vi "niDTS BT BDR Rx Test Example.vi"() -> ()   [LabVIEW 2014]
uses:
  Rx Test/Includes/niDTS BT Rx Test INC Results.ctl
  BDR Rx Test/Includes/niDTS BT BDR Rx Test INC Parameters.ctl
  BDR Tx Test/Includes/niDTS BT INC BDR Packet Type.ctl
  Tx Test/Includes/niDTS BT Tx Test INC BD Payload Data.ctl
  Rx Test/Includes/niDTS BT Rx Test INC Carrier Mode.ctl
  Rx Test/Includes/niDTS BT Rx Test INC Packet Header.ctl
  Rx Test/Includes/niDTS BT Rx Test INC Payload Header.ctl
  Includes/niDTS BT DUT INC SG Trigger.ctl
  CommLib/Includes/niDTS Comm INC CLI Login.ctl
  EDR Rx Test/Includes/niDTS BT EDR Rx Test INC Parameters.ctl
  LE Rx Test/Includes/niDTS BT LE Rx Test INC Parameters.ctl
  Rx Test/Includes/niDTS BT Rx Test INC LE Payload Length.ctl
  Framework/Logger/Includes/niDTS Logger INC File Parameters.ctl
  TestStand/Station/Objects/SystemDutHandle/niDTS SystemDutHandle.lvclass
  Framework/niDTS Framework.lvlib
  TestStand/niDTS TestStand.lvlib
  Plugins/niBCM4350 BT/niBCM4350 BT.lvlib
  niDTS BT.lvlib
  Tx Test/Objects/BASE_class/niDTS BT Tx Test.lvclass
  Rx Test/Objects/BASE_class/niDTS BT Rx Test.lvclass
  Plugins/niLEDTM BT/niLEDTM BT.lvlib
  CommLib/niDTS CommLib.lvlib
panel:
  in  "Result Index":i32=1
  in  "Tab Control":enum32{"BDR", "EDR", "LE TP"}(tab)
  in  "BDR Rx Input Parameters":T1={"Channel"=0, "Tx Power (dBm) "=-70.0, "External Attenuation (dB)"=0.0, "BDR Packet type"=enum."DH1", "Payload Data"=enum."PN9", "Carrier Mode"=enum."Burst", "Number of Packets"=-1, "Report Period (ms)"=1000.0, "BD ADDRESS"="\u0000\u0000\u0000\u0000\u0000\u0000", "Packet Header"={"LT Address"=0, "Flow"=0, "ARQN"=enum."NAK", "Sequence Bit"=0}, "Dirty Packets"=FALSE, "Corrupt Alternate CRC"=FALSE, "Payload Header"={"LCh"=0, "HeaderFlowControlBit"=FALSE, "Length (-1 AutoSet Max)"=-1}, "Trigger"={"TriggerEdge"=enum."RISing", "TriggerSource"=enum."IMMediate", "TriggerDelay (sec)"=0.0, "TriggerTimeout (sec)"=0.0}}
  out "Results":T8
  out "BDR USL":T8={"Total Packets Received (LE)"=2147483647, "Packets Sent (LE)"=inf, "Good Packets"=inf, "Packet Error Rate (%)"=1.0, "Error Bits"=4294967295, "Good Bits"=4294967295, "Total Received Bits"=4294967295, "Bit Error Rate (%)"=1.0}
  out "BDR LSL":T8
  out "EDR USL":T8={"Total Packets Received (LE)"=2147483647, "Packets Sent (LE)"=inf, "Good Packets"=inf, "Packet Error Rate (%)"=1.0, "Error Bits"=4294967295, "Good Bits"=4294967295, "Total Received Bits"=4294967295, "Bit Error Rate (%)"=1.0}
  out "EDR LSL":T8
  out "EDR RX Results":T8
  in  "EDR Rx Input Parameters":T9={"Channel"=0, "Tx Power (dBm)"=-70.0, "External Attenuation (dB)"=0.0, "EDR Packet type"=enum."DH1", "Data Rate (bits/symbol)"=2, "Payload Data"=enum."PN9", "Carrier Mode"=enum."Burst", "Number of Packets"=-1, "Report Period (ms)"=1000.0, "BD ADDRESS"="\u0000\u0000\u0000\u0000\u0000\u0000", "Dirty Packets"=FALSE, "Corrupt Alternate CRC"=FALSE, "Packet Header"={"LT Address"=0, "Flow"=0, "ARQN"=enum."NAK", "Sequence Bit"=0}, "Payload Header"={"LCh"=0, "HeaderFlowControlBit"=FALSE, "Length (-1 AutoSet Max)"=-1}, "Trigger"={"TriggerEdge"=enum."RISing", "TriggerSource"=enum."IMMediate", "TriggerDelay (sec)"=0.0, "TriggerTimeout (sec)"=0.0}}
  out "LE USL":T8={"Total Packets Received (LE)"=2147483647, "Packets Sent (LE)"=inf, "Good Packets"=inf, "Packet Error Rate (%)"=1.0, "Error Bits"=4294967295, "Good Bits"=4294967295, "Total Received Bits"=4294967295, "Bit Error Rate (%)"=1.0}
  out "LE LSL":T8
  out "LE Resutls":T8={"Total Packets Received (LE)"=1500, "Packets Sent (LE)"=1500.0, "Good Packets"=0.0, "Packet Error Rate (%)"=0.0, "Error Bits"=0, "Good Bits"=0, "Total Received Bits"=0, "Bit Error Rate (%)"=0.0}
  in  "BT LE Parameters":T10={"Channel"=0, "Tx Power (dBm)"=-70.0, "External Attenuation (dB)"=0.0, "Payload Data"=enum."PN9", "Carrier Mode"=enum."Burst", "Number of Packets"=1500, "Corrupt Alternate CRC"=FALSE, "Dirty Tx"=FALSE, "Payload Header"={"Length (-1 AutoSet Max)"=-1}, "Trigger"={"TriggerEdge"=enum."RISing", "TriggerSource"=enum."IMMediate", "TriggerDelay (sec)"=0.0, "TriggerTimeout (sec)"=0.0}}
  in  "General Parameters":T13={"Port Parameters Serial"={"baud rate "=115200, "data bits"=8, "Enable Termination Char"=TRUE, "flow control"=0, "parity"=enum."None", "timeout (ms) "=5000, "stop bits"=10, "termination char"=10}, "CLI Login"={"Do Login"=FALSE, "Login Prompt"="", "Password"="", "User Name"=""}}
  in  "Socket Index":i32
  in  "System Configuration Path":path=path "C:/Users/Public/Documents/National Instruments/WTM 1.0/System Configurations/BTDev4_28_2015.xml"
  in  "DUT Plugin":enum32{"LE DTM", "BCM4350"}(tab)=enum."BCM4350"
  in  "Interfaces LE DTM":enum32{"Serial", "Other"}(tab)
  in  "Port Parameters":T14(array[cluster])=[{"BT"={"Serial Resource"="COM5"}}, {"BT"={"Serial Resource"="COM5"}}]
  in  "Interfaces BCM4350":enum32{"Serial", "Other"}(tab)
  in  "Port Parameters":T14(array[cluster])=[{"BT"={"Serial Resource"="COM5"}}, {"BT"={"Serial Resource"="COM5"}}]
  out "error out":errorcluster
  # "BD Address Order"
  # "LAP(24)UAP(8)NAP(16)"
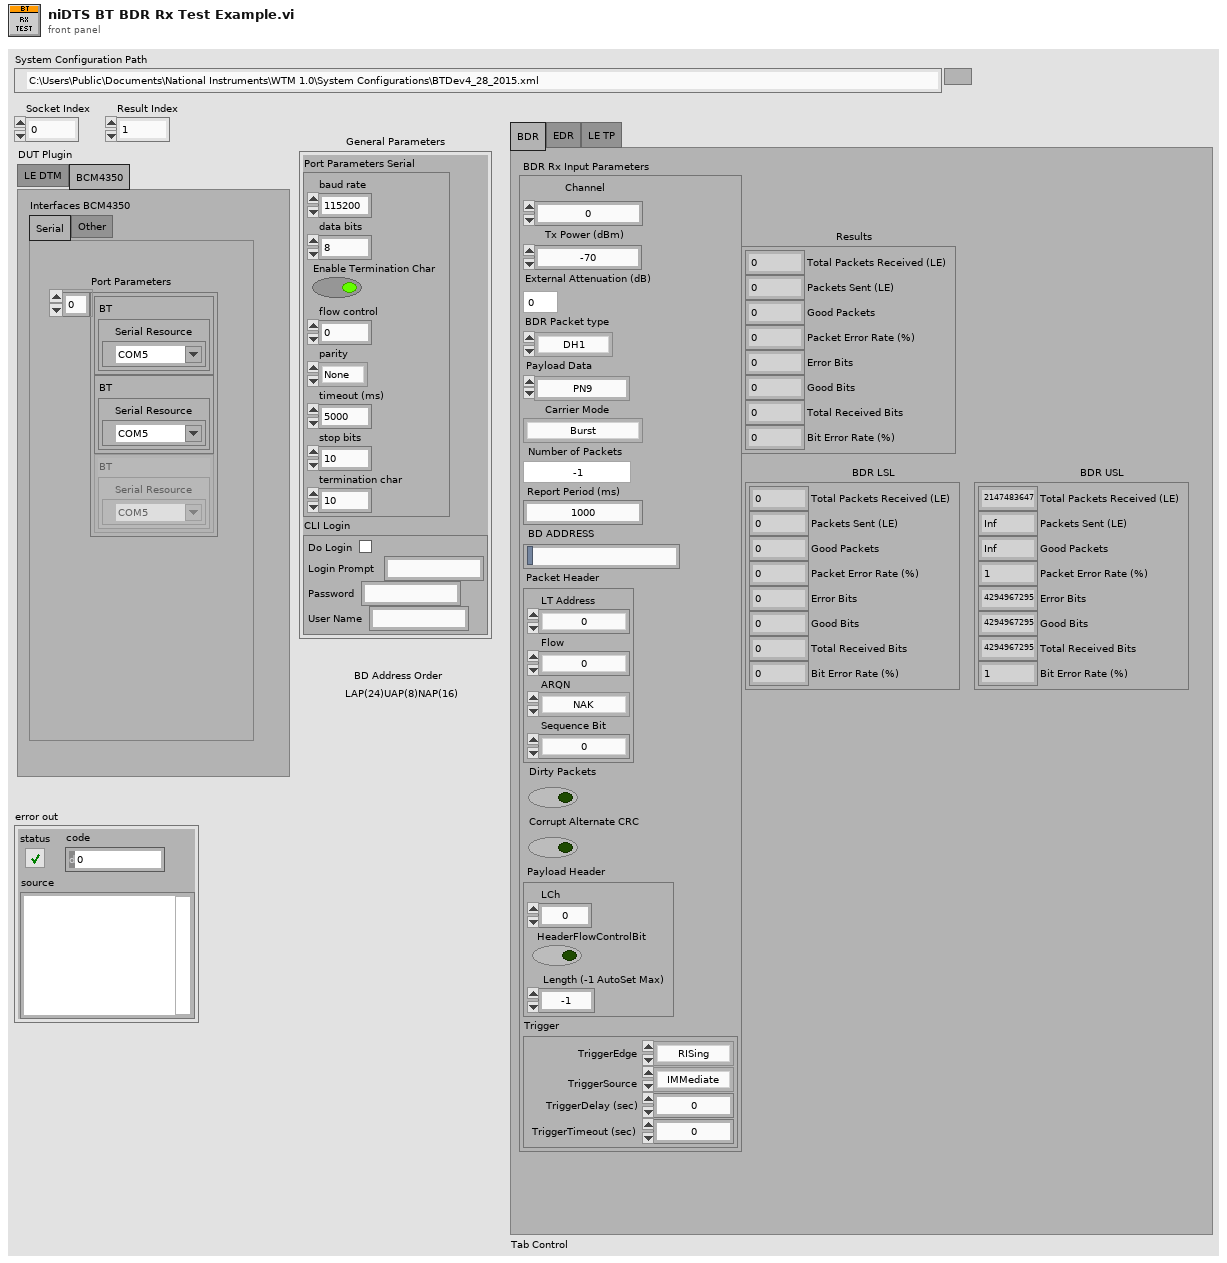
[diagram p1: front panel]
types:
  T1 = typedef "niDTS BT.lvlib/niDTS BT BDR Rx Test INC Parameters.ctl" = cluster{"Channel":i32, "Tx Power (dBm) ":dbl, "External Attenuation (dB)":dbl, "BDR Packet type":T2, "Payload Data":T3, "Carrier Mode":T4, "Number of Packets":i32, "Report Period (ms)":dbl, "BD ADDRESS":string, "Packet Header":T5, "Dirty Packets":bool, "Corrupt Alternate CRC":bool, "Payload Header":T6, "Trigger":T7}
  T2 = typedef "niDTS BT.lvlib/niDTS BT INC BDR Packet Type.ctl" = enum16{"NULL", "POLL", "FHS", "DM1", "DH1", "HV1", "HV2", "HV3", "EV3", "DV", "AUX1", "DM3", "DH3", "EV4", "EV5", "DM5", "DH5"}
  T3 = typedef "niDTS BT.lvlib/niDTS BT Tx Test INC BD Payload Data.ctl" = enum16{"0", "1", "01", "00001111", "PN9", "AUTO"}
  T4 = typedef "niDTS BT.lvlib/niDTS BT Rx Test INC Carrier Mode.ctl" = enum16{"Burst", "Continuous"}
  T5 = typedef "niDTS BT.lvlib/niDTS BT Rx Test INC Packet Header.ctl" = cluster{"LT Address":i8, "Flow":i8, "ARQN":enum16{"NAK", "ACK"}, "Sequence Bit":i8}
  T6 = typedef "niDTS BT.lvlib/niDTS BT Rx Test INC Payload Header.ctl" = cluster{"LCh":i32, "HeaderFlowControlBit":bool, "Length (-1 AutoSet Max)":i32}
  T7 = typedef "niDTS BT.lvlib/niDTS BT DUT INC SG Trigger.ctl" = cluster{"TriggerEdge":enum16{"RISing", "FALLing"}, "TriggerSource":enum16{"IMMediate", "PFI 0", "PFI 1", "RTSI 0", "RTSI 1", "RTSI 2", "RTSI 3", "RTSI 4", "RTSI 5", "RTSI 6", "RTSI 7", "PXI STAR", "Software"}, "TriggerDelay (sec)":dbl, "TriggerTimeout (sec)":dbl}
  T8 = typedef "niDTS BT.lvlib/niDTS BT Rx Test INC Results.ctl" = cluster{"Total Packets Received (LE)":i32, "Packets Sent (LE)":dbl, "Good Packets":dbl, "Packet Error Rate (%)":dbl, "Error Bits":u32, "Good Bits":u32, "Total Received Bits":u32, "Bit Error Rate (%)":dbl}
  T9 = typedef "niDTS BT.lvlib/niDTS BT EDR Rx Test INC Parameters.ctl" = cluster{"Channel":i32, "Tx Power (dBm)":dbl, "External Attenuation (dB)":dbl, "EDR Packet type":T2, "Data Rate (bits/symbol)":i32, "Payload Data":T3, "Carrier Mode":T4, "Number of Packets":i32, "Report Period (ms)":dbl, "BD ADDRESS":string, "Dirty Packets":bool, "Corrupt Alternate CRC":bool, "Packet Header":T5, "Payload Header":T6, "Trigger":T7}
  T10 = typedef "niDTS BT.lvlib/niDTS BT LE Rx Test INC Parameters.ctl" = cluster{"Channel":i32, "Tx Power (dBm)":dbl, "External Attenuation (dB)":dbl, "Payload Data":T3, "Carrier Mode":T4, "Number of Packets":i32, "Corrupt Alternate CRC":bool, "Dirty Tx":bool, "Payload Header":T11, "Trigger":T7}
  T11 = typedef "niDTS BT.lvlib/niDTS BT Rx Test INC LE Payload Length.ctl" = cluster{"Length (-1 AutoSet Max)":i32}
  T12 = typedef "niDTS CommLib.lvlib/niDTS Comm INC CLI Login.ctl" = cluster{"Do Login":bool, "Login Prompt":string, "Password":string, "User Name":string}
  T13 = cluster{"Port Parameters Serial":cluster{"baud rate ":u32, "data bits":u16, "Enable Termination Char":bool, "flow control":u16, "parity":enum16{"None", "Odd", "Even", "Mark", "Space"}, "timeout (ms) ":u32, "stop bits":u16, "termination char":u8}, "CLI Login":T12}
  T14 = cluster{"BT":cluster{"Serial Resource":refnum<visa-resource-name>}}[]
  T15 = typedef "niDTS Framework.lvlib/niDTS Logger INC File Parameters.ctl" = cluster{"File Size (Bytes)":u32, "New File Per Day":bool, "File Location":path, "Base File Name":string}
  T16 = typedef "niDTS Framework.lvlib/niDTS Logger INC Handle.ctl" = refnum<data-value>
  T17 = cluster{"BT":cluster{"Serial Resource":refnum<visa-resource-name>}}
  T18 = typedef "niDTS Framework.lvlib/niDTS Dut INC Handle.ctl" = refnum<data-value>
  T19 = typedef "niDTS BT.lvlib/niDTS BT Rx Test INC Handle.ctl" = refnum<data-value>
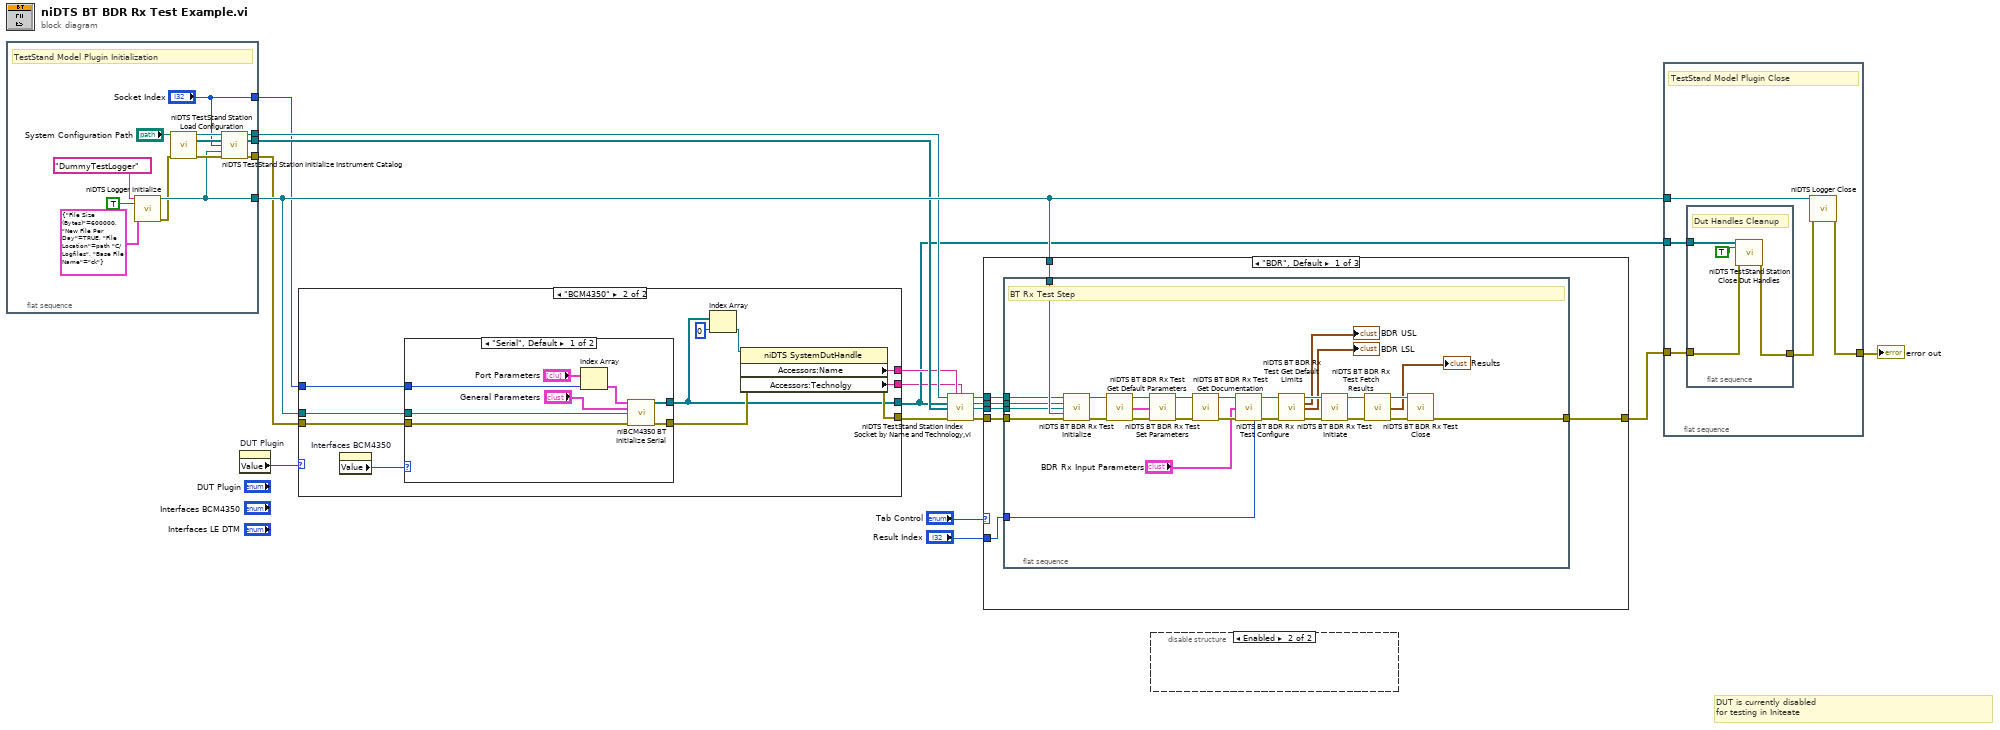
[diagram p0: block diagram]
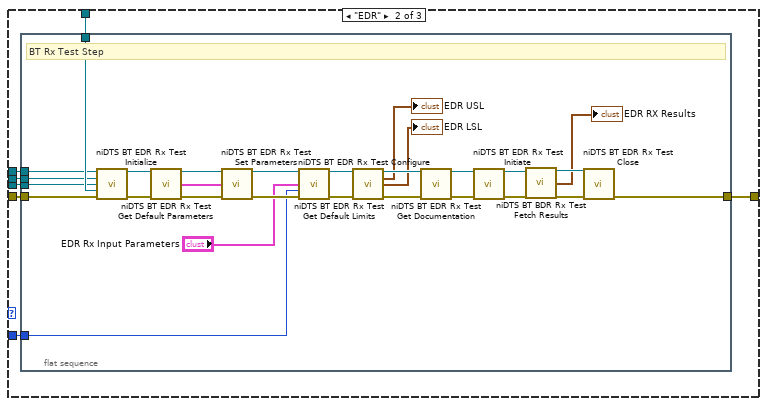
[diagram p2: hidden frame]
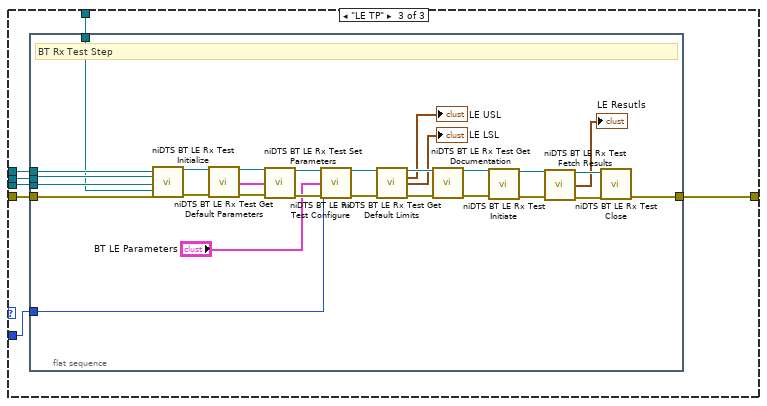
[diagram p3: hidden frame]
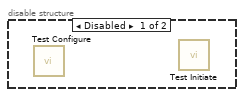
[diagram p4: hidden frame]
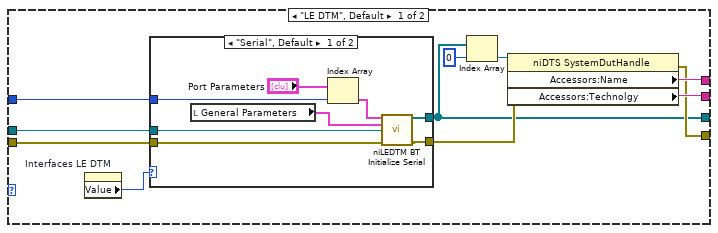
[diagram p5: hidden frame]
diagram:
  # "DUT is currently disabled\nfor testing in Initeate"
  n1 = flat-sequence {
    tunnel: [w26] -> w15
    tunnel: [w23] -> w6
    tunnel: [w22] -> w13
    tunnel: [w24] -> w14
    tunnel: ["Socket Index"] -> w2
    frame #0 {
      # "TestStand Model Plugin Initialization"
      n2 = call "niDTS Logger Initialize.vi"("Session Name ()"="DummyTestLogger", "Log to File"=TRUE, "Logger File Parameters"=T15 {"File Size (Bytes)"=600000, "New File Per Day"=TRUE, "File Location"=path "C:/Logfiles", "Base File Name"="ck"}) -> ("Logger Handle out"=w26:T16, "error out"=w21:errorcluster)  [unwired: 11 in]
      n3 = call "niDTS TestStand Station Load Configuration.vi"("System Configuration XML Path"="System Configuration Path", "error in (no error)"=w21) -> ("All System Hardware"=w29:refnum<class "niDTS SystemHardware.lvclass">, "All DUT Definitions"=w28:refnum<class "niDTS SystemDut.lvclass">[], "error out"=w27:errorcluster)  [unwired: 11 in]
      n4 = call "niDTS TestStand Station Initialize Instrument Catalog.vi"("All System Hardware"=w29, "All DUT Definitions"=w28, "Socket Index"="Socket Index", "Logger Handle"=w26, "error in (no error)"=w27) -> ("Socket Instrument Catalog"=w22:refnum<class "niDTS SystemInstrCatalog.lvclass">, "Socket DUT Definitions"=w24:refnum<class "niDTS SystemDut.lvclass">[], "error out"=w23:errorcluster)  [unwired: 8 in]
    }
  }
  n5 = property on="DUT Plugin" class="TabCtl (strict)"() -> ("Value"=w16:enum32{"LE DTM", "BCM4350"})  [unwired: 2 in, 2 out]
  n6 = case shown="\"BCM4350\"" w16 {
    tunnel: w15 -> [w37 w60]
    tunnel: w6 -> [w36 w61]
    tunnel: [w33 w53] -> w5
    tunnel: [w40 w57] -> w12
    tunnel: [w39 w56] -> w4
    tunnel: [w34 w54] -> w11
    tunnel: w2 -> [w38 w52]
    frame "LE DTM", Default {
      n7 = property on="Interfaces LE DTM" class="TabCtl (strict)"() -> ("Value"=w32:enum32{"Serial", "Other"})  [unwired: 2 in, 2 out]
      n8 = case shown="\"Serial\", Default" w32 {
        tunnel: w38 -> [w49 _]
        tunnel: w37 -> [w48 _]
        tunnel: w36 -> [w47 w51]
        tunnel: [w45 w51] -> w35
        tunnel: [w44 _] -> w33
        frame "Serial", Default {
          n9 = local read "General Parameters"() -> (w46:T13)
          n10 = Index Array(array="Port Parameters", index=w49) -> (element=w50:T17)
          n11 = call "niLEDTM BT Initialize Serial.vi"("Socket Parameters"=w50, "General Parameters"=w46, "Logger"=w48, "error in (no error)"=w47) -> ("DUT Technology Handles"=w44:refnum<class "niDTS SystemDutHandle.lvclass">[], "Error"=w45:errorcluster)  [unwired: 10 in]
        }
        frame "Other" {
          # "Future Implementation"
        }
      }
      n12 = Index Array(array=w33, index=0) -> (element=w41:refnum<class "niDTS SystemDutHandle.lvclass">)
      n13 = property class="niDTS SystemDutHandle"(reference=w41, error in=w35) -> (error out=w34:errorcluster, "Accessors:Name"=w40:string, "Accessors:Technolgy"=w39:string)  [unwired: 1 out]
    }
    frame "BCM4350" {
      n14 = property on="Interfaces BCM4350" class="TabCtl (strict)"() -> ("Value"=w62:enum32{"Serial", "Other"})  [unwired: 2 in, 2 out]
      n15 = case shown="\"Serial\", Default" w62 {
        tunnel: [w67 _] -> w53
        tunnel: [w70 _] -> w55
        tunnel: w61 -> [w69 _]
        tunnel: w60 -> [w68 _]
        tunnel: w52 -> [w63 _]
        frame "Serial", Default {
          n16 = Index Array(array="Port Parameters", index=w63) -> (element=w64:T17)
          n17 = call "niBCM4350 BT Initialize Serial.vi"("Socket Parameters"=w64, "General Parameters"="General Parameters", "Logger"=w68, "error in (no error)"=w69) -> ("DUT Technology Handles"=w67:refnum<class "niDTS SystemDutHandle.lvclass">[], "Error"=w70:errorcluster)  [unwired: 10 in]
        }
        frame "Other" {
          # "Future Implementation"
        }
      }
      n18 = Index Array(array=w53, index=0) -> (element=w58:refnum<class "niDTS SystemDutHandle.lvclass">)
      n19 = property class="niDTS SystemDutHandle"(reference=w58, error in=w55) -> (error out=w54:errorcluster, "Accessors:Name"=w57:string, "Accessors:Technolgy"=w56:string)  [unwired: 1 out]
    }
  }
  n20 = call "niDTS TestStand Station Index Socket by Name and Technology,vi.vi"("niDTS SystemInstrCatalog in"=w13, "Name"=w12, "Technology"=w4, "System Dut Handles"=w5, "Socket DUT Definitions"=w14, "error in (no error)"=w11) -> ("Dut Handle"=w7:T18, "SystemTechnologyCatalog"=w8:refnum<class "niDTS SystemTechnologyCatalog.lvclass">, "Specific Socket/Tech DUT Definition"=w9:refnum<class "niDTS SystemDut.lvclass">, "error out"=w10:errorcluster)  [unwired: 6 in]
  n21 = case shown="\"BDR\", Default" "Tab Control" {
    tunnel: [w77 w112 w147] -> w18
    tunnel: w15 -> [w76 w111 w146]
    tunnel: w10 -> [w75 w110 w145]
    tunnel: w9 -> [w74 w109 w144]
    tunnel: w8 -> [w73 w108 w143]
    tunnel: w7 -> [w72 w107 w142]
    tunnel: "Result Index" -> [w71 w106 w141]
    frame "BDR", Default {
      n22 = flat-sequence {
        tunnel: w76 -> [w95]
        tunnel: [w101] -> w77
        tunnel: w75 -> [w94]
        tunnel: w74 -> [w93]
        tunnel: w73 -> [w92]
        tunnel: w72 -> [w91]
        tunnel: w71 -> [w79]
        frame #0 {
          # "BT Rx Test Step"
          n23 = call "niDTS BT BDR Rx Test  Initialize.vi"("Dut Reference"=w91, "SystemTechnologyCatalog"=w92, "SystemDut"=w93, "Logger Reference"=w95, "error in (no error)"=w94) -> ("RX Test Handle Out"=w84:T19, "error out"=w83:errorcluster)  [unwired: 8 in, 1 out]
          n24 = call "niDTS BT BDR Rx Test Get Default Parameters.vi"("RX Test Handle In"=w84, "error in (no error)"=w83) -> ("RX Test Handle Out"=w86:T19, "BDR Rx Input Parameters"=w81:T1, "error out"=w85:errorcluster)  [unwired: 11 in]
          n25 = call "niDTS BT BDR Rx Test Set Parameters.vi"("RX Test Handle In"=w86, "BT BDR Parameters"=w81, "error in (no error)"=w85) -> ("RX Test Handle Out"=w88:T19, "error out"=w87:errorcluster)  [unwired: 11 in]
          n26 = call "niDTS BT BDR Rx Test Get Documentation.vi"("RX Test Handle In"=w88, "error in (no error)"=w87) -> ("RX Test Handle Out"=w89:T19, "error out"=w90:errorcluster)  [unwired: 11 in, 1 out]
          n27 = call "niDTS BT BDR Rx Test Configure.vi"("Dummy Test Handle In"=w89, "BT BDR Parameters"="BDR Rx Input Parameters", "Result Index"=w79, "error in (no error)"=w90) -> ("Dummy Test Handle Out"=w97:T19, "error out"=w105:errorcluster)  [unwired: 10 in]
          n28 = call "niDTS BT BDR Rx Test Get Default Limits.vi"("Dummy Test Handle In"=w97, "error in (no error)"=w105) -> ("Dummy Test Handle Out"=w104:T19, "USL"=→"BDR USL":T8, "LSL"=→"BDR LSL":T8, "error out"=w78:errorcluster)  [unwired: 10 in]
          n29 = call "niDTS BT BDR Rx Test Initiate.vi"("Dummy Test Handle In"=w104, "error in (no error)"=w78) -> ("Dummy Test Handle Out"=w103:T19, "error out"=w102:errorcluster)  [unwired: 12 in]
          n30 = call "niDTS BT BDR Rx Test Fetch Results.vi"("Dummy Test Handle in"=w103, "error in (no error)"=w102) -> ("Dummy Test Handle out"=w96:T19, "Results"=→"Results":T8, "error out"=w100:errorcluster)  [unwired: 11 in]
          n31 = call "niDTS BT BDR Rx Test Close.vi"("Dummy Test Handle out"=w96, "error in (no error)"=w100) -> ("error out"=w101:errorcluster)  [unwired: 13 in]
        }
      }
    }
    frame "EDR" {
      n32 = flat-sequence {
        tunnel: w111 -> [w139]
        tunnel: [w123] -> w112
        tunnel: w110 -> [w140]
        tunnel: w109 -> [w136]
        tunnel: w108 -> [w137]
        tunnel: w107 -> [w138]
        tunnel: w106 -> [w115]
        frame #0 {
          # "BT Rx Test Step"
          n33 = call "niDTS BT EDR Rx Test  Initialize.vi"("Dut Reference"=w138, "SystemTechnologyCatalog"=w137, "SystemDut"=w136, "Logger Reference"=w139, "error in (no error)"=w140) -> ("RX Test Handle Out"=w134:T19, "error out"=w135:errorcluster)  [unwired: 8 in, 1 out]
          n34 = call "niDTS BT EDR Rx Test Get Default Parameters.vi"("RX Test Handle In"=w134, "error in (no error)"=w135) -> ("RX Test Handle Out"=w133:T19, "EDR  Tx Parameters"=w113:T9, "error out"=w132:errorcluster)  [unwired: 11 in]
          n35 = call "niDTS BT EDR Rx Test Set Parameters.vi"("RX Test Handle"=w133, "Parameters"=w113, "error in (no error)"=w132) -> ("RX Test Handle 2"=w131:T19, "error out"=w130:errorcluster)  [unwired: 11 in]
          n36 = call "niDTS BT EDR Rx Test Configure.vi"("Dummy Test Handle In"=w131, "BT EDR Parameters"="EDR Rx Input Parameters", "Result Index"=w115, "error in (no error)"=w130) -> ("Dummy Test Handle Out"=w129:T19, "error out"=w128:errorcluster)  [unwired: 10 in]
          n37 = call "niDTS BT EDR Rx Test Get Default Limits.vi"("Dummy Test Handle In"=w129, "error in (no error)"=w128) -> ("Dummy Test Handle Out"=w126:T19, "USL"=→"EDR USL":T8, "LSL"=→"EDR LSL":T8, "error out"=w127:errorcluster)  [unwired: 10 in]
          n38 = call "niDTS BT EDR Rx Test Get Documentation.vi"("Dummy Test Handle In"=w126, "error in (no error)"=w127) -> ("Dummy Test Handle Out"=w125:T19, "error out"=w124:errorcluster)  [unwired: 11 in, 1 out]
          n39 = call "niDTS BT EDR Rx Test Initiate.vi"("Dummy Test Handle In"=w125, "error in (no error)"=w124) -> ("Dummy Test Handle Out"=w120:T19, "error out"=w119:errorcluster)  [unwired: 12 in]
          n40 = call "niDTS BT BDR Rx Test Fetch Results.vi"("Dummy Test Handle in"=w120, "error in (no error)"=w119) -> ("Dummy Test Handle out"=w117:T19, "Results"=→"EDR RX Results":T8, "error out"=w118:errorcluster)  [unwired: 11 in]
          n41 = call "niDTS BT EDR Rx Test Close.vi"("Dummy Test Handle out"=w117, "error in (no error)"=w118) -> ("error out"=w123:errorcluster)  [unwired: 13 in]
        }
      }
    }
    frame "LE TP" {
      n42 = flat-sequence {
        tunnel: w146 -> [w172]
        tunnel: [w154] -> w147
        tunnel: w145 -> [w171]
        tunnel: w144 -> [w173]
        tunnel: w143 -> [w174]
        tunnel: w142 -> [w175]
        tunnel: w141 -> [w150]
        frame #0 {
          # "BT Rx Test Step"
          n43 = call "niDTS BT LE Rx Test  Initialize.vi"("Dut Reference"=w175, "SystemTechnologyCatalog"=w174, "SystemDut"=w173, "Logger Reference"=w172, "error in (no error)"=w171) -> ("RX Test Handle Out"=w169:T19, "error out"=w170:errorcluster)  [unwired: 8 in, 1 out]
          n44 = call "niDTS BT LE Rx Test Get Default Parameters.vi"("Dummy Test Handle In"=w169, "error in (no error)"=w170) -> ("Dummy Test Handle Out 2"=w166:T19, "BDR Tx Parameters"=w148:T10, "error out"=w168:errorcluster)  [unwired: 11 in]
          n45 = call "niDTS BT LE Rx Test Set Parameters.vi"("Dummy Test Handle In"=w166, "BT LE Parameters"=w148, "error in (no error)"=w168) -> ("Dummy Test Handle Out"=w165:T19, "error out"=w167:errorcluster)  [unwired: 11 in]
          n46 = call "niDTS BT LE Rx Test Configure.vi"("Dummy Test Handle In"=w165, "BT LE Parameters"="BT LE Parameters", "Result Index"=w150, "error in (no error)"=w167) -> ("Dummy Test Handle Out"=w164:T19, "error out"=w163:errorcluster)  [unwired: 10 in]
          n47 = call "niDTS BT LE Rx Test Get Default Limits.vi"("Dummy Test Handle In"=w164, "error in (no error)"=w163) -> ("Dummy Test Handle Out"=w161:T19, "USL"=→"LE USL":T8, "LSL"=→"LE LSL":T8, "error out"=w162:errorcluster)  [unwired: 10 in]
          n48 = call "niDTS BT LE Rx Test Get Documentation.vi"("Dummy Test Handle In"=w161, "error in (no error)"=w162) -> ("Dummy Test Handle Out"=w160:T19, "error out"=w159:errorcluster)  [unwired: 11 in, 1 out]
          n49 = call "niDTS BT LE Rx Test Initiate.vi"("Dummy Test Handle In"=w160, "error in (no error)"=w159) -> ("Dummy Test Handle Out"=w158:T19, "error out"=w157:errorcluster)  [unwired: 12 in]
          n50 = call "niDTS BT LE Rx Test Fetch Results.vi"("Dummy Test Handle in"=w158, "error in (no error)"=w157) -> ("Dummy Test Handle out"=w156:T19, "Results"=→"LE Resutls":T8, "error out"=w155:errorcluster)  [unwired: 11 in]
          n51 = call "niDTS BT LE Rx Test Close.vi"("Dummy Test Handle out"=w156, "error in (no error)"=w155) -> ("error out"=w154:errorcluster)  [unwired: 13 in]
        }
      }
    }
  }
  n52 = disable-structure shown="Enabled" {
    frame Disabled {
      n53 = call-dynamic "Test Configure.vi"() -> ()  [unwired: 14 in, 2 out]
      n54 = call-dynamic "Test Initiate.vi"() -> ()  [unwired: 14 in, 2 out]
    }
    frame Enabled {
    }
  }
  n55 = flat-sequence {
    tunnel: [w180] -> w17
    tunnel: w15 -> [w179]
    tunnel: w5 -> [w178]
    tunnel: w18 -> [w177]
    frame #0 {
      # "TestStand Model Plugin Close"
      n56 = flat-sequence {
        tunnel: w178 -> [w183]
        tunnel: w177 -> [w182]
        tunnel: [w181] -> w176
        frame #0 {
          # "Dut Handles Cleanup"
          n57 = call "niDTS TestStand Station Close Dut Handles.vi"("Socket Dut Handles In"=w183, "Close All"=TRUE, "error in (no error)"=w182) -> ("error out"=w181:errorcluster)  [unwired: 11 in, 1 out]
        }
      }
      n58 = call "niDTS Logger Close.vi"("Logger Handle in"=w179, "error in (no error)"=w176) -> ("error out"=w180:errorcluster)  [unwired: 13 in]
    }
  }
  "error out" <- w17
